vi "Get_Parameters.vi"(8 "error in (no error)":errorcluster caption="错误输入（无错误）", 11 "Database Command输入":refnum<class "Database Command.lvclass">) -> (0 "error out":errorcluster caption="错误输出", 2 "Parameters":refnum<k7>, 3 "Database Command输出":refnum<class "Database Command.lvclass">)   [LabVIEW 2011, in "Database Command.lvclass"]
uses:
  Database Command.lvclass
  Database Command.lvclass/Database Command.ctl
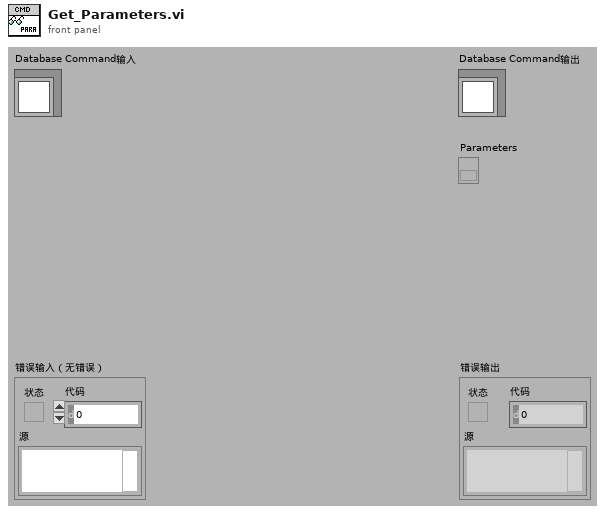
[diagram p1: front panel]
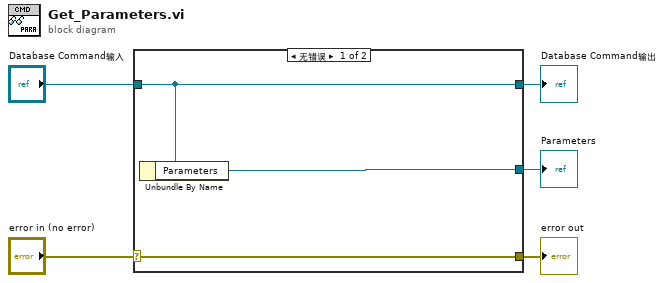
[diagram p0: block diagram]
diagram:
  n1 = case shown="无错误" "error in (no error)" {
    selector: "error in (no error)" -> [w8 w9]
    tunnel: [w8 w9] -> w4
    tunnel: [w7 w10] -> w2
    tunnel: "Database Command输入" -> [w7 w10]
    tunnel: [w6 _] -> w1
    frame No Error {
      n2 = Unbundle By Name(w7) -> ("Parameters"=w6:refnum<k7>)
    }
    frame Error {
    }
  }
  "error out" <- w4
  "Database Command输出" <- w2
  "Parameters" <- w1
